vi "Read Test Listbox.vi"(11 "Test Framework in":refnum<class "Test Framework.lvclass">) -> (0 "Value":i32, 1 "Symbols":i32[](array[numeric]), 2 "Measurement Names":string[](array[string]), 3 "Test Framework out":refnum<class "Test Framework.lvclass">)   [LabVIEW 2020, in "Test Framework.lvclass"]
uses:
  Test Framework.lvclass
  Test Framework.lvclass/Test Framework.ctl
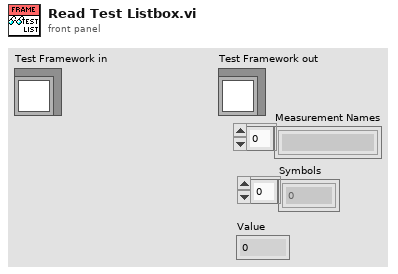
[diagram p1: front panel]
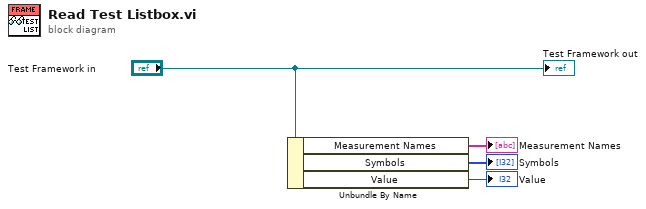
[diagram p0: block diagram]
diagram:
  n1 = Unbundle By Name("Test Framework in") -> ("Measurement Names"=→"Measurement Names":string[], "Symbols"=→"Symbols":i32[], "Value"=→"Value":i32)
  "Test Framework out" <- "Test Framework in"
